vi "saveImage_new2.vi"(4 "error in":errorcluster, 5 "Save reff num":refnum<vi>, 6 "bit depth":enum16{"16bits", "14bits", "12bits", "8bits"}(ring), 7 "pySession in":refnum<k35>, 8 "Reff ROI":T2, 9 "Main ROI":T2, 10 "appended filename":string, 11 "Image In":T1) -> (0 "error out":errorcluster, 3 "png filename":string)   [LabVIEW 2023]
uses:
  <vilib>/vision/Image Controls.llb/IMAQ Image.ctl
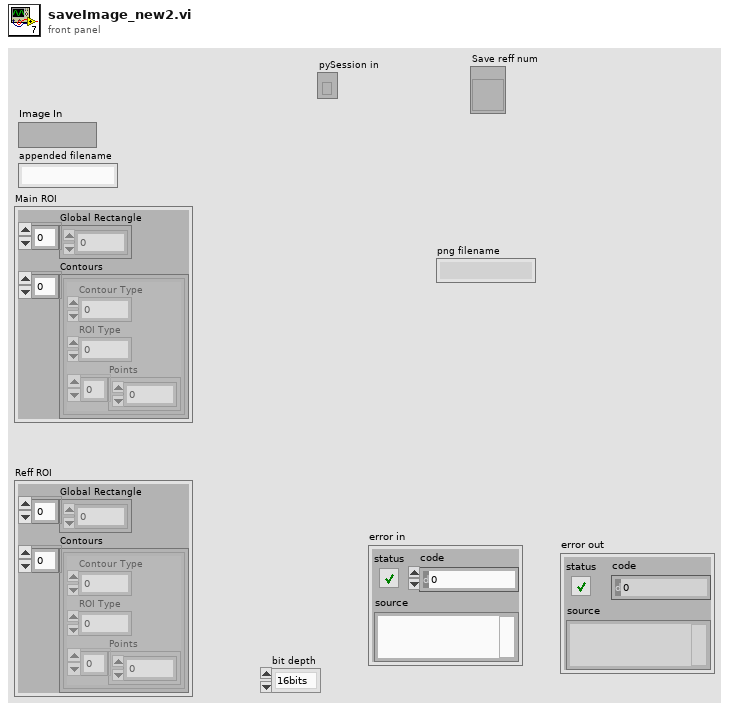
[diagram p1: front panel]
types:
  T1 = typedef "IMAQ Image.ctl" = refnum<image>
  T2 = cluster{"Global Rectangle":i32[], "Contours":cluster{"Contour Type":u32, "ROI Type":u32, "Points":i32[]}[]}
  T3 = enum8{"Enabled", "Disabled", "Disabled and Grayed Out"}
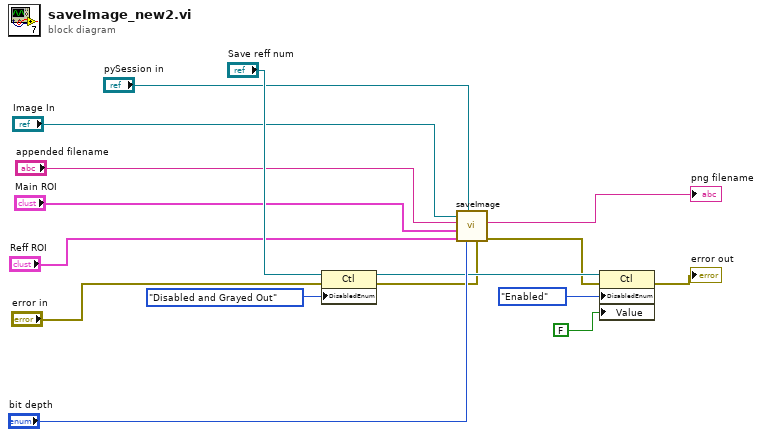
[diagram p0: block diagram]
diagram:
  n1 = property on="Property Node" class="Ctl"(reference="Save reff num", error in="error in", "DisabledEnum"=T3."Disabled and Grayed Out" ("Disabled")) -> (reference out=w8:refnum<vi>, error out=w6:errorcluster)
  n2 = call "saveImage.vi"("error in"=w6, "bit depth"="bit depth", "session in"="pySession in", "Reff ROI"="Reff ROI", "main ROI"="Main ROI", "appended filename"="appended filename", "Image in"="Image In") -> ("error out"=w5:errorcluster, "png filename"=→"png filename":string)  [unwired: 1 in, 2 out]
  n3 = property on="Property Node" class="Ctl"(reference=w8, error in=w5, "DisabledEnum"=T3."Enabled" ("Disabled"), "Value"=FALSE ("Save")) -> (error out=→"error out":errorcluster)  [unwired: 1 out]
